vi "CAN Jaguar Set Voltage Ramp Rate.vi"(8 "error in (no error)":errorcluster, 10 "VoltageRampRate (V/s)":dbl, 11 "CAN Jaguar Ref":T1={"Device Number"=0, "Control Mode"=enum."Percent VBus", "Inverted"=FALSE, "Semaphore"=refnum, "Max Vout"=12.0, "DevStatus"={"status"=FALSE, "code"=0, "source"=""}}) -> (0 "error out":errorcluster, 3 "CAN Jaguar Ref Out":T1={"Device Number"=0, "Control Mode"=enum."Percent VBus", "Inverted"=FALSE, "Semaphore"=refnum, "Max Vout"=12.0, "DevStatus"={"status"=FALSE, "code"=0, "source"=""}})   [LabVIEW 2009, in "CAN.lvlib"]
uses:
  CAN.lvlib
  SubVIs/CAN Jaguar Ref.ctl
  SubVIs/CAN Jaguar Control Mode.ctl
  SubVIs/CAN Motor Message IDs.ctl
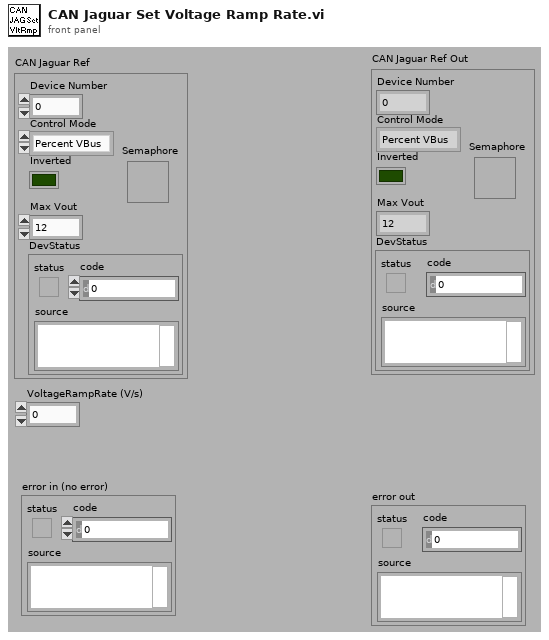
[diagram p1: front panel]
types:
  T1 = typedef "CAN.lvlib/CAN Jaguar Ref.ctl" = cluster{"Device Number":u8, "Control Mode":T2, "Inverted":bool, "Semaphore":T3, "Max Vout":dbl, "DevStatus":errorcluster}
  T2 = typedef "CAN.lvlib/CAN Jaguar Control Mode.ctl" = enum16{"Percent VBus", "Speed", "Position", "Current"}
  T3 = typedef "Semaphore RefNum" = refnum<k1>
  T4 = enum16{"big-endian, network order", "native, host order", "little-endian"}
  T5 = typedef "CAN.lvlib/CAN Motor Message IDs.ctl" = u32
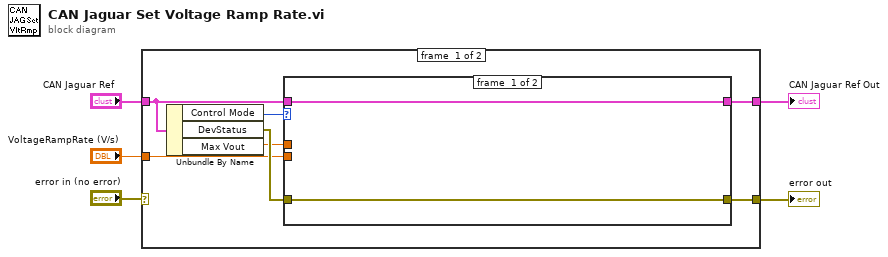
[diagram p0: block diagram]
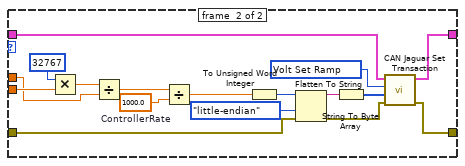
[diagram p2: hidden frame]
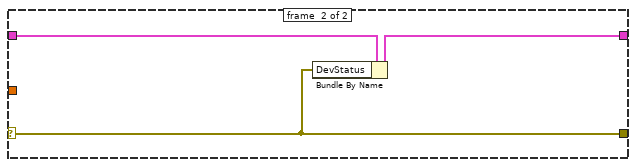
[diagram p3: hidden frame]
diagram:
  n1 = case shown="No Error" "error in (no error)" {
    selector: "error in (no error)" -> [_ w32]
    tunnel: [w8 w32] -> w5
    tunnel: [w7 w33] -> w3
    tunnel: "CAN Jaguar Ref" -> [w9 w34]
    tunnel: "VoltageRampRate (V/s)" -> [w10 _]
    frame #0 {
      n2 = Unbundle By Name(w9) -> ("Control Mode"=w11:T2, "DevStatus"=w12:errorcluster, "Max Vout"=w6:dbl)
      n3 = case shown="\"Percent VBus\"" w11 {
        tunnel: [w14 w16] -> w8
        tunnel: w10 -> [_ w27]
        tunnel: w12 -> [w14 w22]
        tunnel: w9 -> [w13 w21]
        tunnel: [w13 w18] -> w7
        tunnel: w6 -> [_ w15]
        frame #0 {
        }
        frame #1 {
          w28 = 1000.0  # ControllerRate
          w19 = T5 33685696 items=["Volt Enable"=33685504, "Volt Disable"=33685568, "Volt Set"=33685632, "Volt Set Ramp"=33685696, "Speed Enable"=33686528, "Speed Disable"=33686592, "Speed Set"=33686656, "Speed P"=33686720, "Speed I"=33686784, "Speed D"=33686848, "Speed Ref"=33686912, "Position Enable"=33688576, "Position Disable"=33688640, "Position Set"=33688704, "Position P"=33688768, "Position I"=33688832, "Position D"=33688896, "Position Ref"=33688960, "Current Enable"=33689600, "Current Disable"=33689664, "Current Set"=33689728, "Current P"=33689792, "Current I"=33689856, "Current D"=33689920, "Status VOut"=33690624, "Status VBus"=33690688, "Status Current"=33690752, "Status Temp"=33690816, "Status Position"=33690880, "Status Speed"=33690944, "Status Limit"=33691008, "Status Fault"=33691072, "Status Power"=33691136, "Config Num Brushes"=33692672, "Config Encoder Lines"=33692736, "Config Pot Turns"=33692800, "Config Brake Coast"=33692864, "Config Limit Mode"=33692928, "Config Limit Fwd"=33692992, "Config Limit Rev"=33693056, "Config Max VOut"=33693120, "Config Fault Time"=33693184, "Motor Ack"=33693696] ("CAN Motor Message IDs")
          n4 = Multiply(x=u32 32767 ("unsigned 16bit integer"), y=w27) -> (x*y=w25:dbl)
          n5 = Divide(x=w25, y=w15) -> (x/y=w26:dbl)
          n6 = Divide(x=w26, y=w28) -> (x/y=w23:dbl)
          n7 = To Unsigned Word Integer(number=w23) -> (unsigned 16bit integer=w29:u16)
          n8 = Flatten To String(anything=w29, byte order (0:big-endian, network order)=T4."little-endian", error in (no error)=w22) -> (data string=w30:string, error out=w17:errorcluster)  [unwired: 2 out]
          n9 = String To Byte Array(string=w30) -> (unsigned byte array=w20:u8[])
          n10 = call "CAN Jaguar Set Transaction.vi"("error in"=w17, "Data"=w20, "Message ID"=w19, "CAN Jaguar Ref"=w21) -> ("error out"=w16:errorcluster, "CAN Jaguar Ref Out"=w18:T1)  [unwired: 6 out]
        }
      }
    }
    frame #1 {
      n11 = Bundle By Name(cluster=w34, "DevStatus"=w32) -> (w33:T1)
    }
  }
  "CAN Jaguar Ref Out" <- w3
  "error out" <- w5
